vi "Parse IMU Data.vi"(6 "Packet":u8[](array[numeric]), 8 "ID":u8) -> (0 "VerticalSpeedIndicator":picture, 1 "Altitude  (/10000)":dbl, 2 "ArtificialHorizon":picture, 3 "Heading Digital":dbl format="%.1f", 4 "AltitudeIndicator":picture, 5 "CompassGauge":picture, 7 "VerticalSpeedDigital":dbl format="%.1f")   [LabVIEW 2023]
uses:
  SBG Data Cluster.ctl
panel:
  in  "ScaleUnit(F=m; T=feet)":bool
  out "output cluster":T1
  in  "Tab Control":T2(tab)
  out "Up Time":u32
  out "time stamp01":u32
  out "General Status":T3
  out "COM Status":T4
  out "Aiding Status":T5
  out "Clock Status":T6
  out "time stamp02":u32
  out "Year":u16
  out "Month":u8
  out "Day":u8
  out "Hour":u8
  out "Min":u8
  out "Sec":u8
  out "NanoSec":u32
  out "GPS TOW":u32
  out "time stamp03":u32
  out "Filtered Acc-x":sgl
  out "Filtered Acc-y":sgl
  out "Filtered Acc-z":sgl
  out "Filtered Gyro-x":sgl
  out "Filtered Gyro-y":sgl
  out "Filtered Gyro-z":sgl
  out "Temp":sgl
  out "IMU Status":T7
  out "Mag Status":T8
  out "time stamp04":u32
  out "MAG X":sgl
  out "MAG Y":sgl
  out "MAG Z":sgl
  out "ACC X":sgl
  out "ACC Y":sgl
  out "ACC Z":sgl
  out "Yaw":sgl
  out "Pitch":sgl
  out "Roll":sgl
  out "time stamp06":u32
  out "Roll Accuracy":sgl
  out "Yaw Accuracy":sgl
  out "Pitch Accuracy":sgl
  out "Internal Kalman Filter Status":T9
  out "time stamp07":u32
  out "Q0":sgl
  out "Q1":sgl
  out "Q2":sgl
  out "Q3":sgl
  out "Yaw Accuracy":sgl
  out "Pitch Accuracy":sgl
  out "Roll Accuracy":sgl
  out "EKF Latitude":dbl format="%#_16g"
  out "EKF Longitude":dbl format="%#_16g"
  out "EKF Altitude MSL":dbl format="%#_16g"
  out "time stamp08":u32
  out "EKF Velocity N":sgl
  out "EKF Velocity E":sgl
  out "EKF Velocity D":sgl
  out "EKF Velocity N Accuracy":sgl
  out "EKF Velocity E Accuracy":sgl
  out "EKF Velocity D Accuracy":sgl
  out "EKF Latitude Accuracy":sgl
  out "EKF Longitude Accuracy":sgl
  out "EKF Altitude Accuracy":sgl
  out "Undulation":sgl
  out "EKF Altitude WGS-84":dbl format="%#_16g"
  out "Ship Motion Status":T10
  out "Heave Period":sgl
  out "time stamp09":u32
  out "Heave (positive down)":sgl
  out "Surge (positive forward)":sgl
  out "Sway (positive right)":sgl
  out "Longitudinal acceleration (positive forward)":sgl
  out "Lateral acceleration (positive right)":sgl
  out "Vertical acceleration (positive down)":sgl
  out "Longitudinal velocity (positive forward)":sgl
  out "Lateral velocity (positive right)":sgl
  out "Vertical velocity (positive down)":sgl
  out "time stamp13":u32
  out "GPS1 VEL N":sgl
  out "GPS1 VEL E":sgl
  out "GPS1 VEL D":sgl
  out "GPS1 Velocity Status":string
  out "GPS1 VEL N Accuracy":sgl
  out "GPS1 VEL E Accuracy":sgl
  out "GPS1 VEL D Accuracy":sgl
  out "GPS1 TOW":u32
  out "GPS1 Course":sgl
  out "GPS1 Course Accuracy":sgl
  out "GPS1 Velocity Type":string
  out "time stamp14":u32
  out "GPS1 Base Station ID":u16
  out "GPS1 Differential Data age":u16
  out "GPS1 Altitude WGS-84 2":dbl
  out "GPS1 POS Status":string
  out "GPS1 POS Type":string
  out "GPS1 POS TOW":u32
  out "GPS1 Latitude":dbl format="%#_16g"
  out "GPS1 Longitude":dbl format="%#_16g"
  out "GPS1 Altitude MSL":dbl
  out "GPS1 Undulation":sgl
  out "GPS1 Latitude Accuracy":sgl
  out "GPS1 Longitude Accuracy":sgl
  out "GPS1 Altitude Accuracy":sgl
  out "GPS1 SV_NUM":u8
  out "GPS1 Status":T11
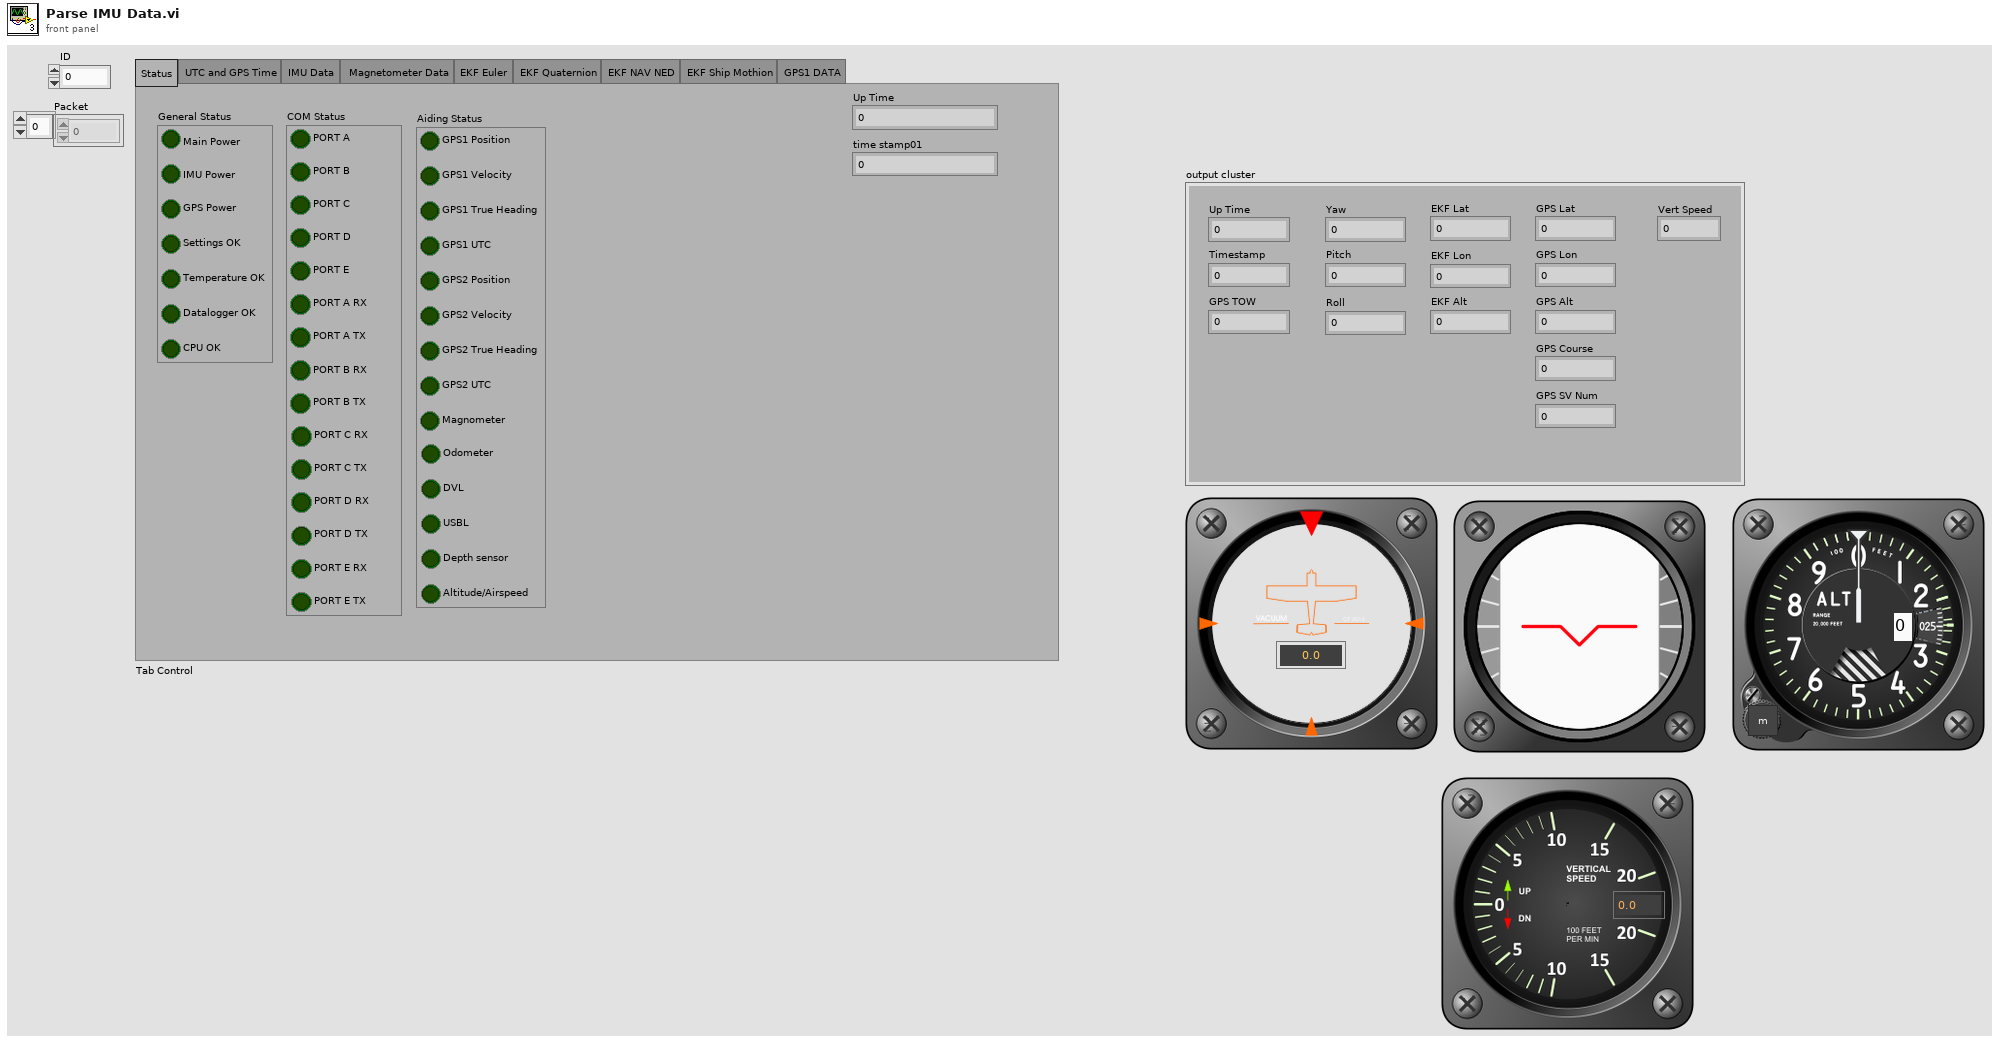
[diagram p1: front panel]
types:
  T1 = typedef "SBG Data Cluster.ctl" = cluster{"Up Time":u32, "Timestamp":u32, "Yaw":sgl, "Pitch":sgl, "Roll":sgl, "EKF Lat":dbl, "EKF Lon":dbl, "EKF Alt":dbl, "GPS Lat":dbl, "GPS Lon":dbl, "GPS Alt":dbl, "GPS Course":sgl, "GPS SV Num":u8, "GPS TOW":u32, "Vert Speed":dbl}
  T2 = enum32{"Status", "UTC and GPS Time", "IMU Data", "Magnetometer Data ", "EKF Euler", "EKF Quaternion", "EKF NAV NED", "EKF Ship Mothion", "GPS1 DATA"}
  T3 = cluster{"Main Power":bool, "IMU Power":bool, "GPS Power":bool, "Settings OK":bool, "Temperature OK":bool, "Datalogger OK":bool, "CPU OK":bool}
  T4 = cluster{"PORT A":bool, "PORT B":bool, "PORT C":bool, "PORT D":bool, "PORT E":bool, "PORT A RX":bool, "PORT A TX":bool, "PORT B RX":bool, "PORT B TX":bool, "PORT C RX":bool, "PORT C TX":bool, "PORT D RX":bool, "PORT D TX":bool, "PORT E RX":bool, "PORT E TX":bool}
  T5 = cluster{"GPS1 Position":bool, "GPS1 Velocity":bool, "GPS1 True Heading":bool, "GPS1 UTC":bool, "GPS2 Position":bool, "GPS2 Velocity":bool, "GPS2 True Heading":bool, "GPS2 UTC":bool, "Magnometer":bool, "Odometer":bool, "DVL":bool, "USBL":bool, "Depth sensor":bool, "Altitude/Airspeed":bool}
  T6 = cluster{"Clock Stable":bool, "Clock Error":bool, "Free Running":bool, "Steering":bool, "Valid and converged":bool, "UTC Sync":bool, "UTC Invalid":bool, "UTC no leap sec":bool, "UTC Valid":bool}
  T7 = cluster{"IMU COM":bool, "IMU BIT":bool, "ACC X BIT":bool, "ACC Y BIT":bool, "ACC Z BIT":bool, "GYRO X BIT":bool, "GYRO Y BIT":bool, "GYTO Z BIT":bool, "ACC  Range":bool, "GYRO Range":bool}
  T8 = cluster{"MAG X BIT":bool, "MAG Y BIT":bool, "MAG Z BIT":bool, "MAG ACC X BIT":bool, "MAG ACC Y BIT":bool, "MAG ACC Z BIT":bool, "MAG Range":bool, "MAG ACC Range":bool, "MAG Calibration":bool}
  T9 = cluster{"Mode Unintialized":bool, "Mode Vertical Gyro":bool, "Mode AHRS":bool, "Mode NAV_VEL":bool, "Attitude":bool, "Heading":bool, "Velocity":bool, "Position":bool, "Vertical Ref Used":bool, "MAG Ref Used":bool, "GPS1 VEL Used":bool, "GPS1 POS Used":bool, "Boolean array[25]":bool, "GPS1 HDT Used":bool, "GPS2 VEL Used":bool, "GPS2 POS Used":bool, "Boolean array[26]":bool, "GPS2 HDT Used":bool, "Odometer Used":bool, "DVL BT Used":bool, "DVL WT Used":bool, "Boolean array[28]":bool, "Boolean array[27]":bool, "Boolean array[28] 2":bool, "USBL Used":bool, "Air Data Used":bool, "ZUPT Used":bool, "Align Used":bool, "Depth Used":bool}
  T10 = cluster{"Heave Valid":bool, "VEL Aided":bool, "Surge Sway Included":bool, "Period Included":bool, "Period Valid":bool, "Swell Mode":bool}
  T11 = cluster{"GPS L1":bool, "GPS L2":bool, "GPS L5":bool, "GLONASS L1":bool, "GLONASS L2":bool, "GLONASS L3":bool, "Galileo E1":bool, "Galileo E5a":bool, "Galileo E5b":bool, "Galileo E5":bool, "Galileo E6":bool, "BeiDou B1":bool, "BeiDou B2":bool, "BeiDou B3":bool, "QZSS L1CA":bool, "QZSS L2C":bool, "QZSS L5":bool}
  T12 = enum16{"GPS Altitude", "Baro absolute Altitude", "Baro Vario"}
  T13 = cluster{"Boolean array[0]":bool, "Boolean array[1]":bool, "Boolean array[2]":bool, "Boolean array[3]":bool, "Boolean array[4]":bool, "Boolean array[5]":bool, "Boolean array[6]":bool, "Boolean array[7]":bool, "Boolean array[8]":bool, "Boolean array[9]":bool, "Boolean array[10]":bool, "Boolean array[11]":bool, "Boolean array[12]":bool, "Boolean array[13]":bool, "Boolean array[14]":bool}
  T14 = cluster{"Boolean array[0]":bool, "Boolean array[1]":bool, "Boolean array[2]":bool, "Boolean array[3]":bool, "Boolean array[4]":bool, "Boolean array[5]":bool, "Boolean array[6]":bool, "Boolean array[7]":bool, "Boolean array[8]":bool, "Boolean array[9]":bool, "Boolean array[10]":bool, "Boolean array[11]":bool, "Boolean array[12]":bool, "Boolean array[13]":bool}
  T15 = cluster{"Boolean array[0]":bool, "Boolean array[1]":bool, "Boolean array[2]":bool, "Boolean array[3]":bool, "Boolean array[4]":bool, "Boolean array[5]":bool, "Boolean array[6]":bool}
  T16 = cluster{"Boolean array[0]":bool, "Boolean array[1]":bool, "Boolean array[2]":bool, "Boolean array[3]":bool, "Boolean array[4]":bool, "Boolean array[5]":bool, "Boolean array[6]":bool, "Boolean array[7]":bool, "Boolean array[8]":bool}
  T17 = cluster{"Boolean array[0]":bool, "Boolean array[1]":bool, "Boolean array[2]":bool, "Boolean array[3]":bool, "Boolean array[4]":bool, "Boolean array[5]":bool, "Boolean array[6]":bool, "Boolean array[7]":bool, "Boolean array[8]":bool, "Boolean array[9]":bool}
  T18 = cluster{"Boolean array[0]":bool, "Boolean array[1]":bool, "Boolean array[2]":bool, "Boolean array[3]":bool, "Boolean array[4]":bool, "Boolean array[5]":bool, "Boolean array[6]":bool, "Boolean array[7]":bool, "Boolean array[8]":bool, "Boolean array[9]":bool, "Boolean array[10]":bool, "Boolean array[11]":bool, "Boolean array[12]":bool, "Boolean array[13]":bool, "Boolean array[14]":bool, "Boolean array[15]":bool, "Boolean array[16]":bool, "Boolean array[17]":bool, "Boolean array[18]":bool, "Boolean array[19]":bool, "Boolean array[20]":bool, "Boolean array[21]":bool, "Boolean array[22]":bool, "Boolean array[23]":bool, "Boolean array[24]":bool, "Boolean array[25]":bool, "Boolean array[26]":bool, "Boolean array[27]":bool, "Boolean array[28]":bool}
  T19 = cluster{"Boolean array[0]":bool, "Boolean array[1]":bool, "Boolean array[2]":bool, "Boolean array[3]":bool, "Boolean array[4]":bool, "Boolean array[5]":bool}
  T20 = cluster{"Boolean array[0]":bool, "Boolean array[1]":bool, "Boolean array[2]":bool, "Boolean array[3]":bool, "Boolean array[4]":bool, "Boolean array[5]":bool, "Boolean array[6]":bool, "Boolean array[7]":bool, "Boolean array[8]":bool, "Boolean array[9]":bool, "Boolean array[10]":bool, "Boolean array[11]":bool, "Boolean array[12]":bool, "Boolean array[13]":bool, "Boolean array[14]":bool, "Boolean array[15]":bool, "Boolean array[16]":bool}
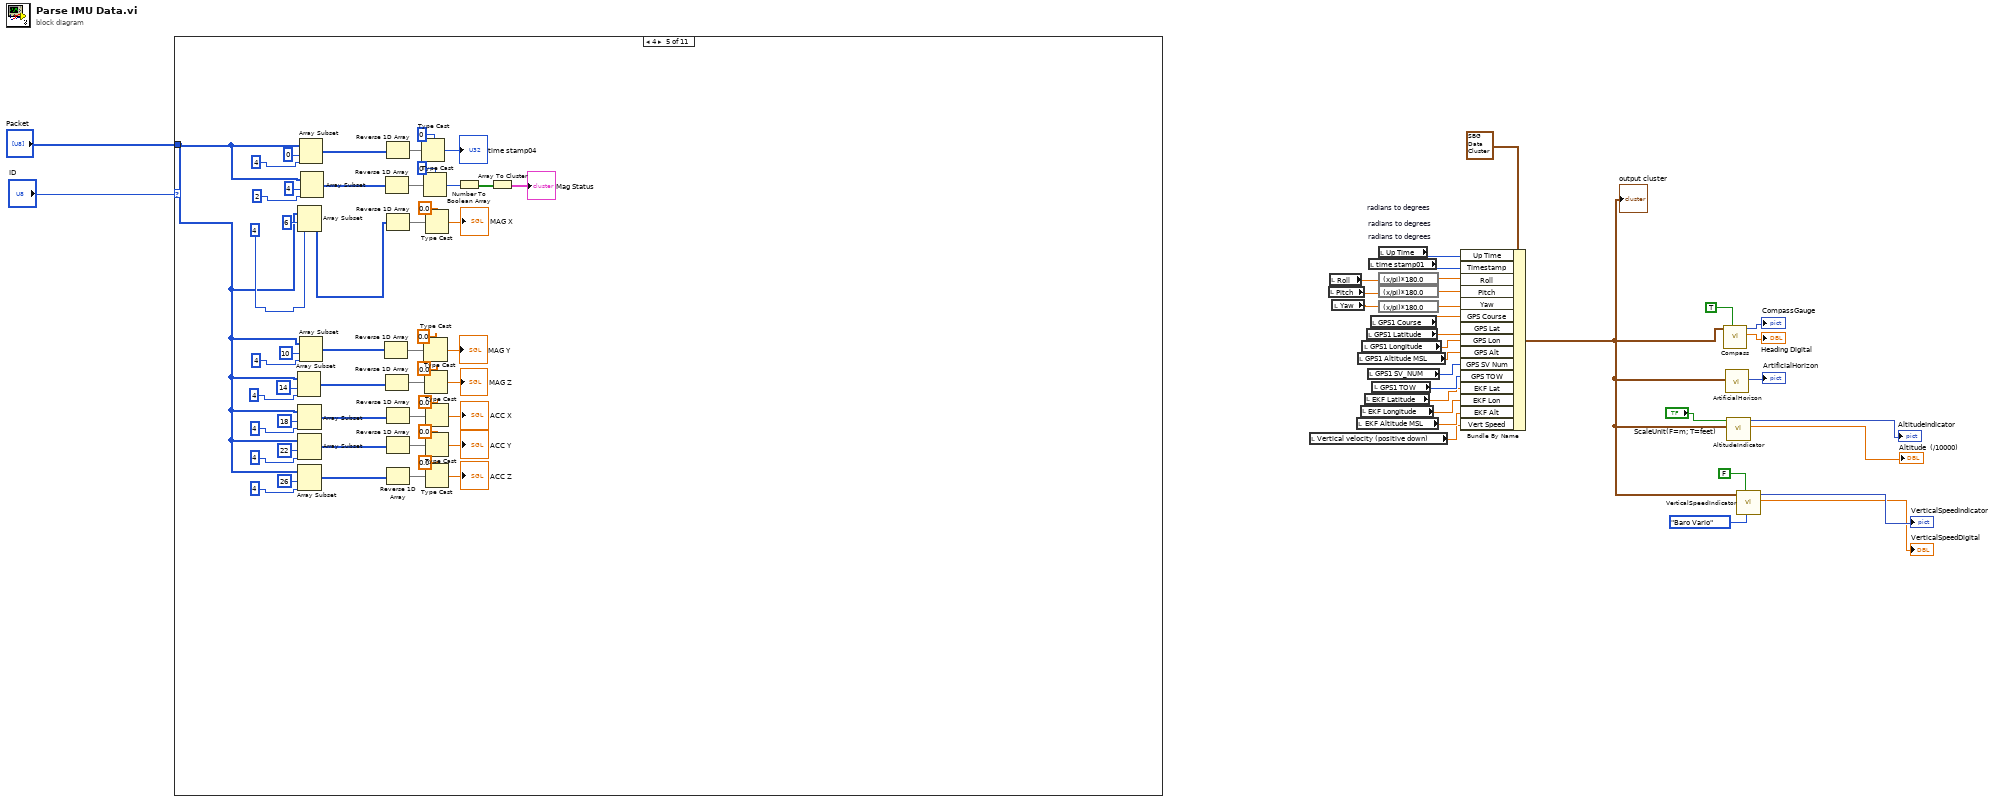
[diagram p0: block diagram]
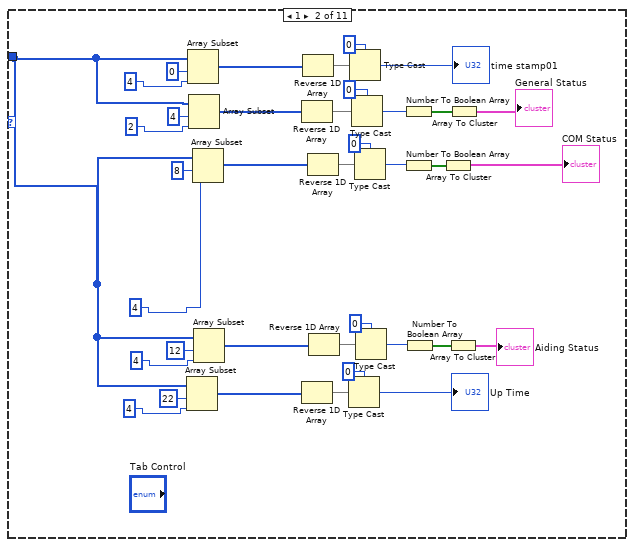
[diagram p3: hidden frame]
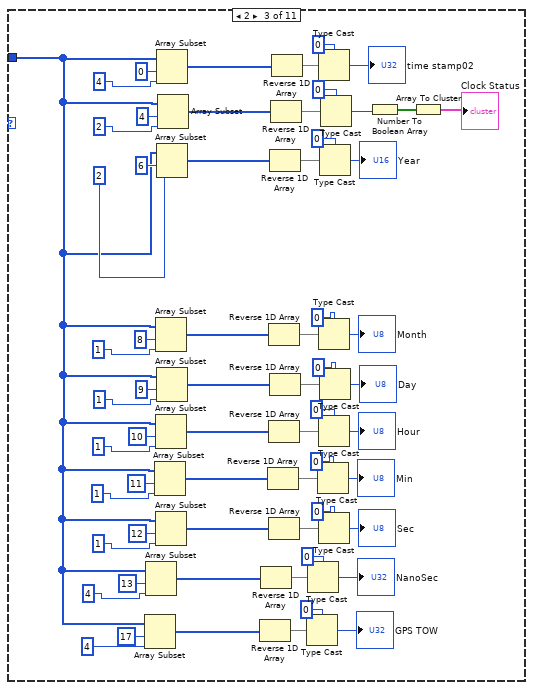
[diagram p4: hidden frame]
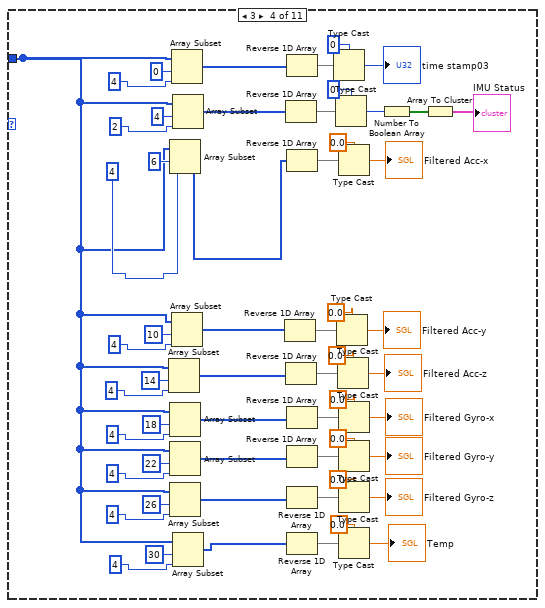
[diagram p5: hidden frame]
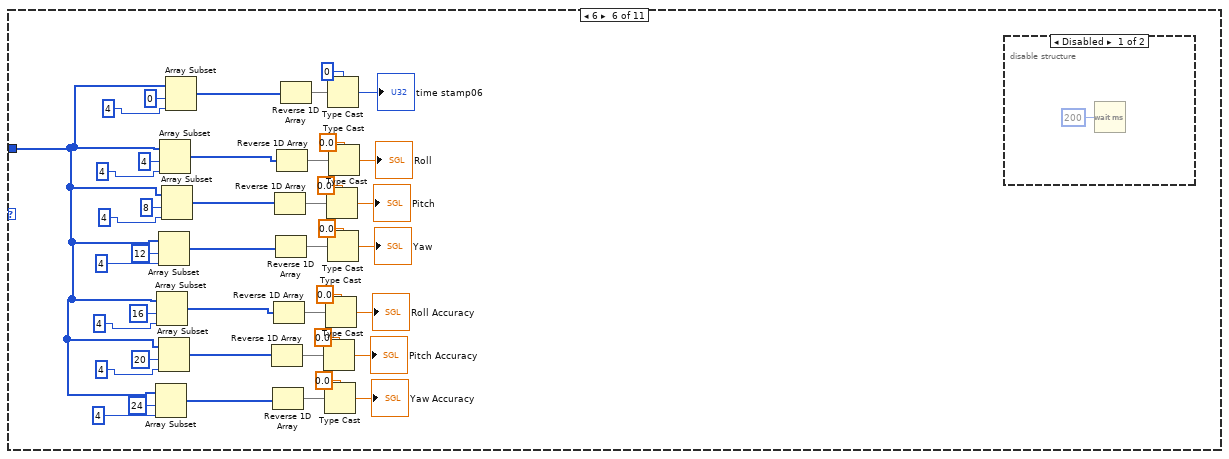
[diagram p6: hidden frame]
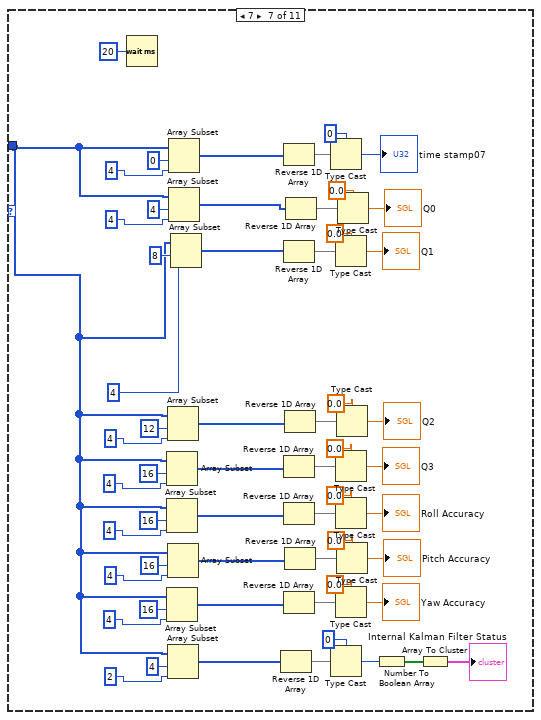
[diagram p8: hidden frame]
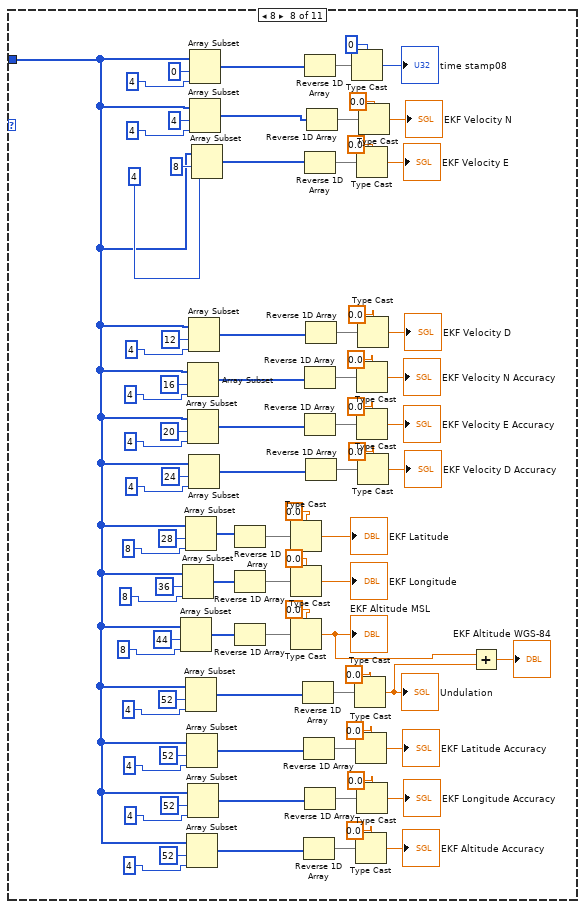
[diagram p9: hidden frame]
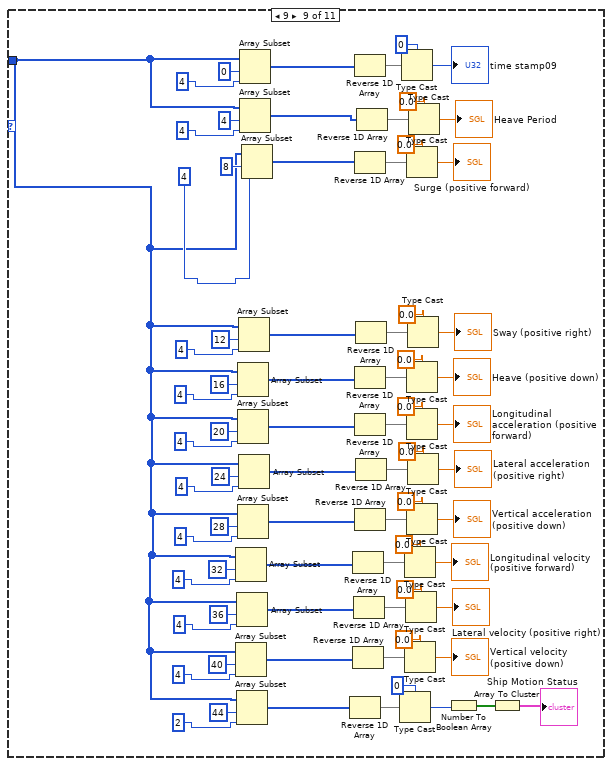
[diagram p10: hidden frame]
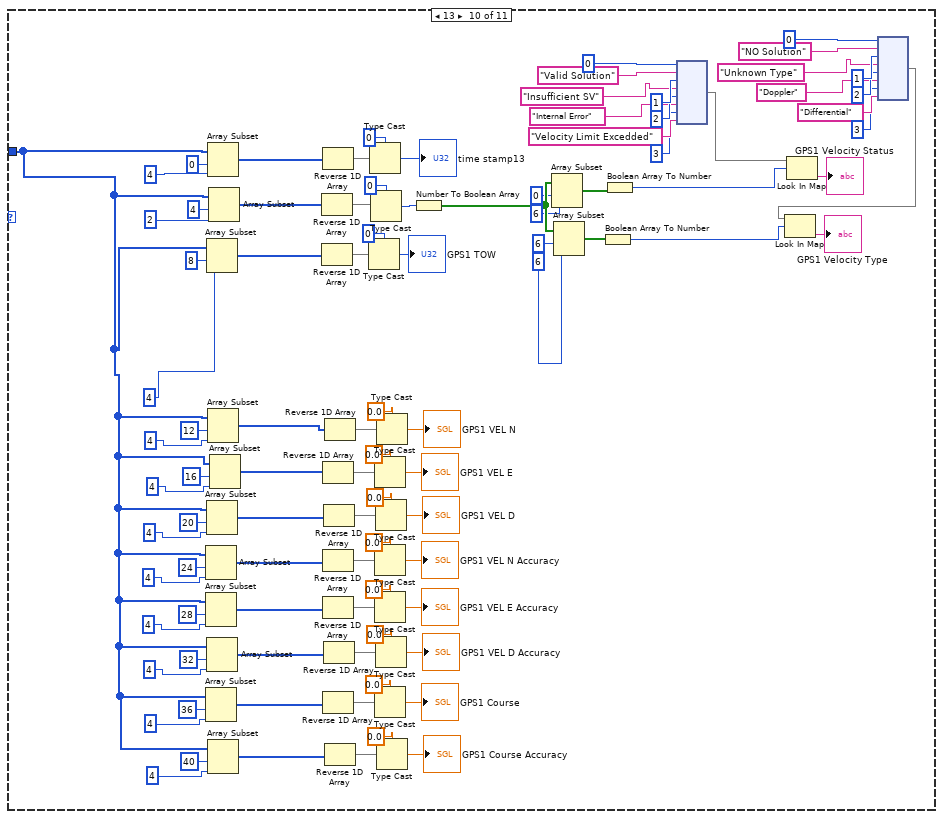
[diagram p11: hidden frame]
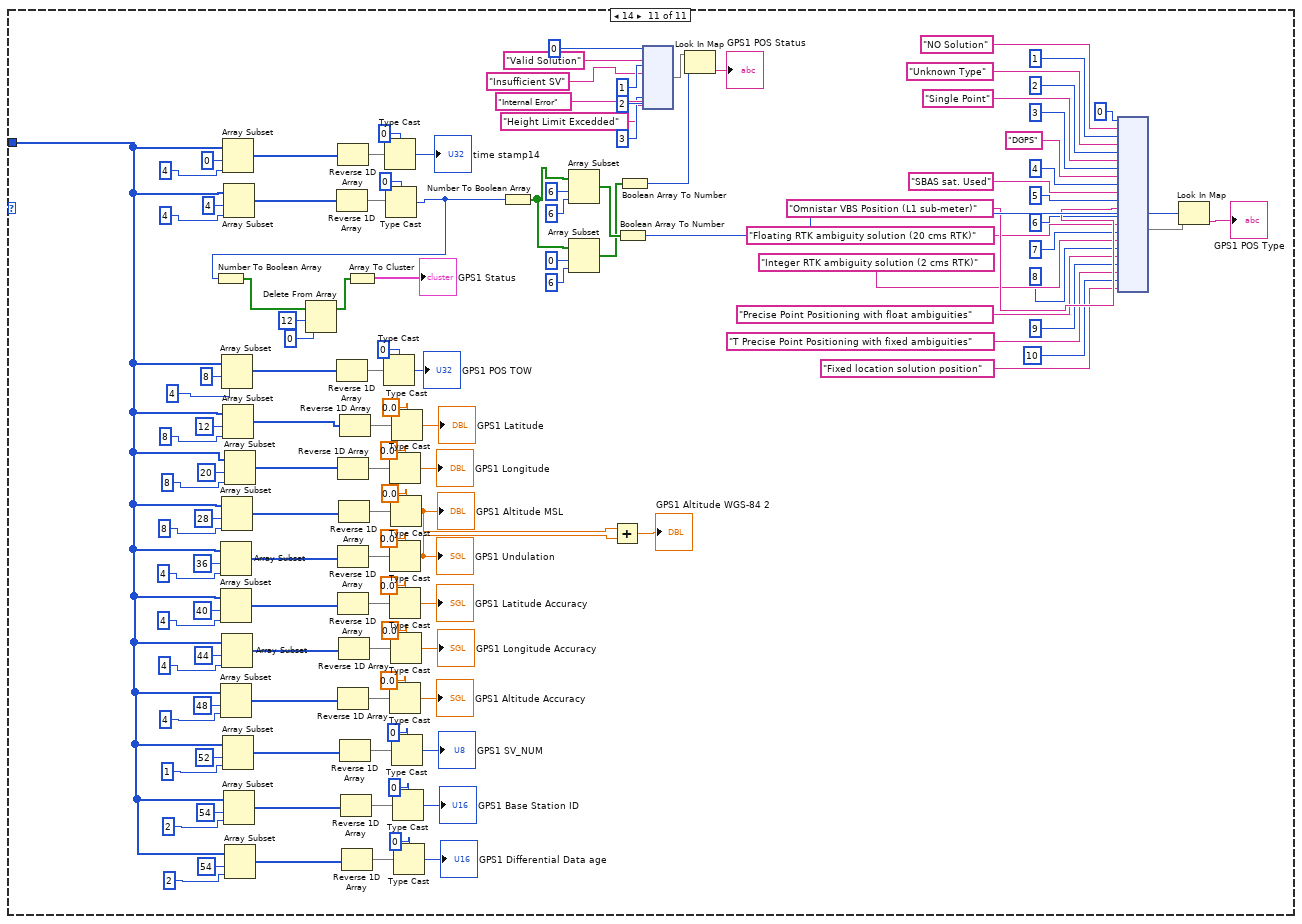
[diagram p12: hidden frame]
diagram:
  n1 = case shown="4" "ID" {
    tunnel: "Packet" -> [_ w37 w71 w137 w191 w246 w287 w344 w430 w539 w610]
    frame 0, Default {
    }
    frame 1 {
      n2 = Array Subset(array=w37, index=22, length=4) -> (w39:u8[])
      n3 = Array Subset(array=w37, index=0, length=4) -> (w68:u8[])
      n4 = Array Subset(array=w37, index=4, length=2) -> (w66:u8[])
      n5 = Array Subset(array=w37, index=8, length=4) -> (w54:u8[])
      n6 = Array Subset(array=w37, index=12, length=4) -> (w47:u8[])
      n7 = Reverse 1D Array(array=w66) -> (reversed array=w70:u8[])
      n8 = Reverse 1D Array(array=w39) -> (reversed array=w38:u8[])
      n9 = Reverse 1D Array(array=w68) -> (reversed array=w69:u8[])
      n10 = Reverse 1D Array(array=w54) -> (reversed array=w53:u8[])
      n11 = Reverse 1D Array(array=w47) -> (reversed array=w48:u8[])
      n12 = Type Cast(type=u32 0, x=w38) -> (*(type *) &x=→"Up Time":u32)
      n13 = Type Cast(type=u32 0, x=w69) -> (*(type *) &x=→"time stamp01":u32)
      n14 = Type Cast(type=u16 0, x=w70) -> (*(type *) &x=w59:u16)
      n15 = Type Cast(type=u32 0, x=w53) -> (*(type *) &x=w52:u32)
      n16 = Type Cast(type=u32 0, x=w48) -> (*(type *) &x=w49:u32)
      n17 = Number To Boolean Array(number=w59) -> (Boolean array=w58:bool[])
      n18 = Number To Boolean Array(number=w52) -> (Boolean array=w51:bool[])
      n19 = Number To Boolean Array(number=w49) -> (Boolean array=w50:bool[])
      n20 = Array To Cluster(array=w51) -> (cluster=→"COM Status":T13)
      n21 = Array To Cluster(array=w50) -> (cluster=→"Aiding Status":T14)
      n22 = Array To Cluster(array=w58) -> (cluster=→"General Status":T15)
    }
    frame 2 {
      n23 = Array Subset(array=w71, index=17, length=4) -> (w73:u8[])
      n24 = Array Subset(array=w71, index=13, length=4) -> (w82:u8[])
      n25 = Array Subset(array=w71, index=11, length=1) -> (w94:u8[])
      n26 = Array Subset(array=w71, index=8, length=1) -> (w109:u8[])
      n27 = Array Subset(array=w71, index=10, length=1) -> (w85:u8[])
      n28 = Array Subset(array=w71, index=12, length=1) -> (w97:u8[])
      n29 = Array Subset(array=w71, index=0, length=4) -> (w125:u8[])
      n30 = Array Subset(array=w71, index=6, length=2) -> (w118:u8[])
      n31 = Array Subset(array=w71, index=9, length=1) -> (w106:u8[])
      n32 = Array Subset(array=w71, index=4, length=2) -> (w128:u8[])
      n33 = Reverse 1D Array(array=w73) -> (reversed array=w72:u8[])
      n34 = Reverse 1D Array(array=w82) -> (reversed array=w83:u8[])
      n35 = Reverse 1D Array(array=w94) -> (reversed array=w95:u8[])
      n36 = Reverse 1D Array(array=w109) -> (reversed array=w108:u8[])
      n37 = Reverse 1D Array(array=w85) -> (reversed array=w84:u8[])
      n38 = Reverse 1D Array(array=w97) -> (reversed array=w96:u8[])
      n39 = Reverse 1D Array(array=w118) -> (reversed array=w119:u8[])
      n40 = Reverse 1D Array(array=w106) -> (reversed array=w107:u8[])
      n41 = Reverse 1D Array(array=w128) -> (reversed array=w123:u8[])
      n42 = Reverse 1D Array(array=w125) -> (reversed array=w124:u8[])
      n43 = Type Cast(type=u32 0, x=w72) -> (*(type *) &x=→"GPS TOW":u32)
      n44 = Type Cast(type=u32 0, x=w83) -> (*(type *) &x=→"NanoSec":u32)
      n45 = Type Cast(type=u8 0, x=w95) -> (*(type *) &x=→"Min":u8)
      n46 = Type Cast(type=u32 0, x=w124) -> (*(type *) &x=→"time stamp02":u32)
      n47 = Type Cast(type=u8 0, x=w108) -> (*(type *) &x=→"Month":u8)
      n48 = Type Cast(type=u8 0, x=w84) -> (*(type *) &x=→"Hour":u8)
      n49 = Type Cast(type=u8 0, x=w96) -> (*(type *) &x=→"Sec":u8)
      n50 = Type Cast(type=u16 0, x=w119) -> (*(type *) &x=→"Year":u16)
      n51 = Type Cast(type=u8 0, x=w107) -> (*(type *) &x=→"Day":u8)
      n52 = Type Cast(type=u16 0, x=w123) -> (*(type *) &x=w120:u16)
      n53 = Number To Boolean Array(number=w120) -> (Boolean array=w122:bool[])
      n54 = Array To Cluster(array=w122) -> (cluster=→"Clock Status":T16)
    }
    frame 3 {
      n55 = Array Subset(array=w137, index=14, length=4) -> (w156:u8[])
      n56 = Array Subset(array=w137, index=6, length=4) -> (w164:u8[])
      n57 = Array Subset(array=w137, index=18, length=4) -> (w155:u8[])
      n58 = Array Subset(array=w137, index=22, length=4) -> (w144:u8[])
      n59 = Array Subset(array=w137, index=26, length=4) -> (w143:u8[])
      n60 = Array Subset(array=w137, index=0, length=4) -> (w171:u8[])
      n61 = Array Subset(array=w137, index=10, length=4) -> (w160:u8[])
      n62 = Array Subset(array=w137, index=4, length=2) -> (w174:u8[])
      n63 = Array Subset(array=w137, index=30, length=4) -> (w176:u8[])
      n64 = Reverse 1D Array(array=w160) -> (reversed array=w163:u8[])
      n65 = Reverse 1D Array(array=w174) -> (reversed array=w168:u8[])
      n66 = Reverse 1D Array(array=w156) -> (reversed array=w157:u8[])
      n67 = Reverse 1D Array(array=w171) -> (reversed array=w169:u8[])
      n68 = Reverse 1D Array(array=w164) -> (reversed array=w165:u8[])
      n69 = Reverse 1D Array(array=w155) -> (reversed array=w154:u8[])
      n70 = Reverse 1D Array(array=w144) -> (reversed array=w145:u8[])
      n71 = Reverse 1D Array(array=w143) -> (reversed array=w142:u8[])
      n72 = Reverse 1D Array(array=w176) -> (reversed array=w170:u8[])
      n73 = Type Cast(type=u32 0, x=w169) -> (*(type *) &x=→"time stamp03":u32)
      n74 = Type Cast(type=u16 0, x=w168) -> (*(type *) &x=w134:u16)
      n75 = Type Cast(type=sgl 0.0, x=w163) -> (*(type *) &x=→"Filtered Acc-y":sgl)
      n76 = Type Cast(type=sgl 0.0, x=w157) -> (*(type *) &x=→"Filtered Acc-z":sgl)
      n77 = Type Cast(type=sgl 0.0, x=w165) -> (*(type *) &x=→"Filtered Acc-x":sgl)
      n78 = Type Cast(type=sgl 0.0, x=w154) -> (*(type *) &x=→"Filtered Gyro-x":sgl)
      n79 = Type Cast(type=sgl 0.0, x=w145) -> (*(type *) &x=→"Filtered Gyro-y":sgl)
      n80 = Type Cast(type=sgl 0.0, x=w142) -> (*(type *) &x=→"Filtered Gyro-z":sgl)
      n81 = Type Cast(type=sgl 0.0, x=w170) -> (*(type *) &x=→"Temp":sgl)
      n82 = Number To Boolean Array(number=w134) -> (Boolean array=w136:bool[])
      n83 = Array To Cluster(array=w136) -> (cluster=→"IMU Status":T17)
    }
    frame 4 {
      n84 = Array Subset(array=w191, index=14, length=4) -> (w213:u8[])
      n85 = Array Subset(array=w191, index=6, length=4) -> (w221:u8[])
      n86 = Array Subset(array=w191, index=18, length=4) -> (w212:u8[])
      n87 = Array Subset(array=w191, index=22, length=4) -> (w201:u8[])
      n88 = Array Subset(array=w191, index=26, length=4) -> (w200:u8[])
      n89 = Array Subset(array=w191, index=0, length=4) -> (w227:u8[])
      n90 = Array Subset(array=w191, index=10, length=4) -> (w217:u8[])
      n91 = Array Subset(array=w191, index=4, length=2) -> (w230:u8[])
      n92 = Reverse 1D Array(array=w217) -> (reversed array=w220:u8[])
      n93 = Reverse 1D Array(array=w230) -> (reversed array=w225:u8[])
      n94 = Reverse 1D Array(array=w213) -> (reversed array=w214:u8[])
      n95 = Reverse 1D Array(array=w227) -> (reversed array=w226:u8[])
      n96 = Reverse 1D Array(array=w221) -> (reversed array=w222:u8[])
      n97 = Reverse 1D Array(array=w212) -> (reversed array=w211:u8[])
      n98 = Reverse 1D Array(array=w201) -> (reversed array=w202:u8[])
      n99 = Reverse 1D Array(array=w200) -> (reversed array=w199:u8[])
      n100 = Type Cast(type=u32 0, x=w226) -> (*(type *) &x=→"time stamp04":u32)
      n101 = Type Cast(type=u16 0, x=w225) -> (*(type *) &x=w192:u16)
      n102 = Type Cast(type=sgl 0.0, x=w220) -> (*(type *) &x=→"MAG Y":sgl)
      n103 = Type Cast(type=sgl 0.0, x=w214) -> (*(type *) &x=→"MAG Z":sgl)
      n104 = Type Cast(type=sgl 0.0, x=w222) -> (*(type *) &x=→"MAG X":sgl)
      n105 = Type Cast(type=sgl 0.0, x=w211) -> (*(type *) &x=→"ACC X":sgl)
      n106 = Type Cast(type=sgl 0.0, x=w202) -> (*(type *) &x=→"ACC Y":sgl)
      n107 = Type Cast(type=sgl 0.0, x=w199) -> (*(type *) &x=→"ACC Z":sgl)
      n108 = Number To Boolean Array(number=w192) -> (Boolean array=w194:bool[])
      n109 = Array To Cluster(array=w194) -> (cluster=→"Mag Status":T16)
    }
    frame 6 {
      n110 = Array Subset(array=w246, index=24, length=4) -> (w252:u8[])
      n111 = Array Subset(array=w246, index=16, length=4) -> (w260:u8[])
      n112 = Array Subset(array=w246, index=12, length=4) -> (w270:u8[])
      n113 = Array Subset(array=w246, index=20, length=4) -> (w256:u8[])
      n114 = Array Subset(array=w246, index=4, length=4) -> (w276:u8[])
      n115 = Array Subset(array=w246, index=8, length=4) -> (w273:u8[])
      n116 = Array Subset(array=w246, index=0, length=4) -> (w248:u8[])
      n117 = Reverse 1D Array(array=w256) -> (reversed array=w259:u8[])
      n118 = Reverse 1D Array(array=w252) -> (reversed array=w253:u8[])
      n119 = Reverse 1D Array(array=w260) -> (reversed array=w261:u8[])
      n120 = Reverse 1D Array(array=w273) -> (reversed array=w275:u8[])
      n121 = Reverse 1D Array(array=w270) -> (reversed array=w271:u8[])
      n122 = Reverse 1D Array(array=w276) -> (reversed array=w277:u8[])
      n123 = Reverse 1D Array(array=w248) -> (reversed array=w247:u8[])
      n124 = Type Cast(type=sgl 0.0, x=w259) -> (*(type *) &x=→"Pitch Accuracy":sgl)
      n125 = Type Cast(type=sgl 0.0, x=w253) -> (*(type *) &x=→"Yaw Accuracy":sgl)
      n126 = Type Cast(type=sgl 0.0, x=w261) -> (*(type *) &x=→"Roll Accuracy":sgl)
      n127 = Type Cast(type=sgl 0.0, x=w275) -> (*(type *) &x=→"Pitch":sgl)
      n128 = Type Cast(type=u32 0, x=w247) -> (*(type *) &x=→"time stamp06":u32)
      n129 = Type Cast(type=sgl 0.0, x=w271) -> (*(type *) &x=→"Yaw":sgl)
      n130 = Type Cast(type=sgl 0.0, x=w277) -> (*(type *) &x=→"Roll":sgl)
      n131 = disable-structure shown="Disabled" {
        frame Disabled {
          n132 = Wait (ms)(milliseconds to wait=u32 200) -> ()  [unwired: 1 out]
        }
        frame Enabled {
        }
      }
    }
    frame 7 {
      n133 = Wait (ms)(milliseconds to wait=u32 20) -> ()  [unwired: 1 out]
      n134 = Array Subset(array=w287, index=16, length=4) -> (w319:u8[])
      n135 = Array Subset(array=w287, index=16, length=4) -> (w308:u8[])
      n136 = Array Subset(array=w287, index=16, length=4) -> (w296:u8[])
      n137 = Array Subset(array=w287, index=12, length=4) -> (w326:u8[])
      n138 = Array Subset(array=w287, index=16, length=4) -> (w307:u8[])
      n139 = Array Subset(array=w287, index=4, length=2) -> (w292:u8[])
      n140 = Array Subset(array=w287, index=0, length=4) -> (w324:u8[])
      n141 = Array Subset(array=w287, index=4, length=4) -> (w334:u8[])
      n142 = Array Subset(array=w287, index=8, length=4) -> (w330:u8[])
      n143 = Reverse 1D Array(array=w292) -> (reversed array=w291:u8[])
      n144 = Reverse 1D Array(array=w324) -> (reversed array=w325:u8[])
      n145 = Reverse 1D Array(array=w330) -> (reversed array=w333:u8[])
      n146 = Reverse 1D Array(array=w319) -> (reversed array=w318:u8[])
      n147 = Reverse 1D Array(array=w308) -> (reversed array=w309:u8[])
      n148 = Reverse 1D Array(array=w296) -> (reversed array=w297:u8[])
      n149 = Reverse 1D Array(array=w326) -> (reversed array=w327:u8[])
      n150 = Reverse 1D Array(array=w307) -> (reversed array=w306:u8[])
      n151 = Reverse 1D Array(array=w334) -> (reversed array=w335:u8[])
      n152 = Type Cast(type=u32 0, x=w325) -> (*(type *) &x=→"time stamp07":u32)
      n153 = Type Cast(type=u16 0, x=w291) -> (*(type *) &x=w288:u16)
      n154 = Type Cast(type=sgl 0.0, x=w333) -> (*(type *) &x=→"Q1":sgl)
      n155 = Type Cast(type=sgl 0.0, x=w318) -> (*(type *) &x=→"Q3":sgl)
      n156 = Type Cast(type=sgl 0.0, x=w309) -> (*(type *) &x=→"Roll Accuracy":sgl)
      n157 = Type Cast(type=sgl 0.0, x=w297) -> (*(type *) &x=→"Yaw Accuracy":sgl)
      n158 = Type Cast(type=sgl 0.0, x=w327) -> (*(type *) &x=→"Q2":sgl)
      n159 = Type Cast(type=sgl 0.0, x=w306) -> (*(type *) &x=→"Pitch Accuracy":sgl)
      n160 = Type Cast(type=sgl 0.0, x=w335) -> (*(type *) &x=→"Q0":sgl)
      n161 = Number To Boolean Array(number=w288) -> (Boolean array=w290:bool[])
      n162 = Array To Cluster(array=w290) -> (cluster=→"Internal Kalman Filter Status":T18)
    }
    frame 8 {
      n163 = Array Subset(array=w344, index=44, length=8) -> (w415:u8[])
      n164 = Array Subset(array=w344, index=36, length=8) -> (w416:u8[])
      n165 = Array Subset(array=w344, index=28, length=8) -> (w423:u8[])
      n166 = Array Subset(array=w344, index=52, length=4) -> (w366:u8[])
      n167 = Array Subset(array=w344, index=52, length=4) -> (w361:u8[])
      n168 = Array Subset(array=w344, index=52, length=4) -> (w349:u8[])
      n169 = Array Subset(array=w344, index=16, length=4) -> (w388:u8[])
      n170 = Array Subset(array=w344, index=20, length=4) -> (w377:u8[])
      n171 = Array Subset(array=w344, index=52, length=4) -> (w352:u8[])
      n172 = Array Subset(array=w344, index=12, length=4) -> (w395:u8[])
      n173 = Array Subset(array=w344, index=24, length=4) -> (w376:u8[])
      n174 = Array Subset(array=w344, index=0, length=4) -> (w393:u8[])
      n175 = Array Subset(array=w344, index=4, length=4) -> (w403:u8[])
      n176 = Array Subset(array=w344, index=8, length=4) -> (w399:u8[])
      n177 = Reverse 1D Array(array=w423) -> (reversed array=w421:u8[])
      n178 = Reverse 1D Array(array=w416) -> (reversed array=w414:u8[])
      n179 = Reverse 1D Array(array=w415) -> (reversed array=w413:u8[])
      n180 = Type Cast(type=0.0, x=w421) -> (*(type *) &x=→"EKF Latitude":dbl)
      n181 = Type Cast(type=0.0, x=w414) -> (*(type *) &x=→"EKF Longitude":dbl)
      n182 = Type Cast(type=0.0, x=w413) -> (*(type *) &x=w365:dbl)
      "EKF Altitude MSL" <- w365
      n183 = Reverse 1D Array(array=w366) -> (reversed array=w367:u8[])
      n184 = Reverse 1D Array(array=w361) -> (reversed array=w360:u8[])
      n185 = Reverse 1D Array(array=w349) -> (reversed array=w348:u8[])
      n186 = Reverse 1D Array(array=w393) -> (reversed array=w394:u8[])
      n187 = Reverse 1D Array(array=w399) -> (reversed array=w402:u8[])
      n188 = Reverse 1D Array(array=w388) -> (reversed array=w387:u8[])
      n189 = Reverse 1D Array(array=w377) -> (reversed array=w378:u8[])
      n190 = Reverse 1D Array(array=w352) -> (reversed array=w353:u8[])
      n191 = Reverse 1D Array(array=w395) -> (reversed array=w396:u8[])
      n192 = Reverse 1D Array(array=w376) -> (reversed array=w375:u8[])
      n193 = Reverse 1D Array(array=w403) -> (reversed array=w404:u8[])
      n194 = Type Cast(type=u32 0, x=w394) -> (*(type *) &x=→"time stamp08":u32)
      n195 = Type Cast(type=sgl 0.0, x=w367) -> (*(type *) &x=w364:sgl)
      "Undulation" <- w364
      n196 = Type Cast(type=sgl 0.0, x=w360) -> (*(type *) &x=→"EKF Latitude Accuracy":sgl)
      n197 = Type Cast(type=sgl 0.0, x=w348) -> (*(type *) &x=→"EKF Altitude Accuracy":sgl)
      n198 = Type Cast(type=sgl 0.0, x=w402) -> (*(type *) &x=→"EKF Velocity E":sgl)
      n199 = Type Cast(type=sgl 0.0, x=w387) -> (*(type *) &x=→"EKF Velocity N Accuracy":sgl)
      n200 = Type Cast(type=sgl 0.0, x=w378) -> (*(type *) &x=→"EKF Velocity E Accuracy":sgl)
      n201 = Type Cast(type=sgl 0.0, x=w353) -> (*(type *) &x=→"EKF Longitude Accuracy":sgl)
      n202 = Type Cast(type=sgl 0.0, x=w396) -> (*(type *) &x=→"EKF Velocity D":sgl)
      n203 = Type Cast(type=sgl 0.0, x=w375) -> (*(type *) &x=→"EKF Velocity D Accuracy":sgl)
      n204 = Type Cast(type=sgl 0.0, x=w404) -> (*(type *) &x=→"EKF Velocity N":sgl)
      n205 = Add(x=w365, y=w364) -> (x+y=→"EKF Altitude WGS-84":dbl)
    }
    frame 9 {
      n206 = Array Subset(array=w430, index=32, length=4) -> (w446:u8[])
      n207 = Array Subset(array=w430, index=40, length=4) -> (w455:u8[])
      n208 = Array Subset(array=w430, index=36, length=4) -> (w445:u8[])
      n209 = Array Subset(array=w430, index=44, length=2) -> (w435:u8[])
      n210 = Array Subset(array=w430, index=16, length=4) -> (w496:u8[])
      n211 = Array Subset(array=w430, index=20, length=4) -> (w501:u8[])
      n212 = Array Subset(array=w430, index=28, length=4) -> (w462:u8[])
      n213 = Array Subset(array=w430, index=12, length=4) -> (w492:u8[])
      n214 = Array Subset(array=w430, index=24, length=4) -> (w502:u8[])
      n215 = Array Subset(array=w430, index=0, length=4) -> (w494:u8[])
      n216 = Array Subset(array=w430, index=4, length=4) -> (w486:u8[])
      n217 = Array Subset(array=w430, index=8, length=4) -> (w489:u8[])
      n218 = Reverse 1D Array(array=w435) -> (reversed array=w434:u8[])
      n219 = Reverse 1D Array(array=w446) -> (reversed array=w447:u8[])
      n220 = Reverse 1D Array(array=w455) -> (reversed array=w456:u8[])
      n221 = Reverse 1D Array(array=w445) -> (reversed array=w444:u8[])
      n222 = Reverse 1D Array(array=w494) -> (reversed array=w493:u8[])
      n223 = Reverse 1D Array(array=w489) -> (reversed array=w487:u8[])
      n224 = Reverse 1D Array(array=w496) -> (reversed array=w497:u8[])
      n225 = Reverse 1D Array(array=w501) -> (reversed array=w500:u8[])
      n226 = Reverse 1D Array(array=w462) -> (reversed array=w461:u8[])
      n227 = Reverse 1D Array(array=w492) -> (reversed array=w491:u8[])
      n228 = Reverse 1D Array(array=w502) -> (reversed array=w503:u8[])
      n229 = Reverse 1D Array(array=w486) -> (reversed array=w485:u8[])
      n230 = Type Cast(type=u16 0, x=w434) -> (*(type *) &x=w431:u16)
      n231 = Type Cast(type=u32 0, x=w493) -> (*(type *) &x=→"time stamp09":u32)
      n232 = Type Cast(type=sgl 0.0, x=w447) -> (*(type *) &x=→"Longitudinal velocity (positive forward)":sgl)
      n233 = Type Cast(type=sgl 0.0, x=w456) -> (*(type *) &x=→"Vertical velocity (positive down)":sgl)
      n234 = Type Cast(type=sgl 0.0, x=w444) -> (*(type *) &x=→"Lateral velocity (positive right)":sgl)
      n235 = Type Cast(type=sgl 0.0, x=w487) -> (*(type *) &x=→"Surge (positive forward)":sgl)
      n236 = Type Cast(type=sgl 0.0, x=w497) -> (*(type *) &x=→"Heave (positive down)":sgl)
      n237 = Type Cast(type=sgl 0.0, x=w500) -> (*(type *) &x=→"Longitudinal acceleration (positive forward)":sgl)
      n238 = Type Cast(type=sgl 0.0, x=w461) -> (*(type *) &x=→"Vertical acceleration (positive down)":sgl)
      n239 = Type Cast(type=sgl 0.0, x=w491) -> (*(type *) &x=→"Sway (positive right)":sgl)
      n240 = Type Cast(type=sgl 0.0, x=w503) -> (*(type *) &x=→"Lateral acceleration (positive right)":sgl)
      n241 = Type Cast(type=sgl 0.0, x=w485) -> (*(type *) &x=→"Heave Period":sgl)
      n242 = Number To Boolean Array(number=w431) -> (Boolean array=w433:bool[])
      n243 = Array To Cluster(array=w433) -> (cluster=→"Ship Motion Status":T19)
    }
    frame 13 {
      n244 = Array Subset(array=w539, index=24, length=4) -> (w578:u8[])
      n245 = Array Subset(array=w539, index=28, length=4) -> (w583:u8[])
      n246 = Array Subset(array=w539, index=36, length=4) -> (w550:u8[])
      n247 = Array Subset(array=w539, index=8, length=4) -> (w599:u8[])
      n248 = Array Subset(array=w539, index=20, length=4) -> (w577:u8[])
      n249 = Array Subset(array=w539, index=32, length=4) -> (w584:u8[])
      n250 = Array Subset(array=w539, index=0, length=4) -> (w597:u8[])
      n251 = Array Subset(array=w539, index=12, length=4) -> (w571:u8[])
      n252 = Array Subset(array=w539, index=40, length=4) -> (w541:u8[])
      n253 = Array Subset(array=w539, index=4, length=2) -> (w596:u8[])
      n254 = Array Subset(array=w539, index=16, length=4) -> (w574:u8[])
      n255 = Reverse 1D Array(array=w596) -> (reversed array=w533:u8[])
      n256 = Reverse 1D Array(array=w599) -> (reversed array=w600:u8[])
      n257 = Reverse 1D Array(array=w597) -> (reversed array=w598:u8[])
      n258 = Reverse 1D Array(array=w574) -> (reversed array=w572:u8[])
      n259 = Reverse 1D Array(array=w578) -> (reversed array=w579:u8[])
      n260 = Reverse 1D Array(array=w583) -> (reversed array=w582:u8[])
      n261 = Reverse 1D Array(array=w550) -> (reversed array=w549:u8[])
      n262 = Reverse 1D Array(array=w577) -> (reversed array=w576:u8[])
      n263 = Reverse 1D Array(array=w584) -> (reversed array=w585:u8[])
      n264 = Reverse 1D Array(array=w571) -> (reversed array=w570:u8[])
      n265 = Reverse 1D Array(array=w541) -> (reversed array=w542:u8[])
      n266 = Type Cast(type=u32 0, x=w600) -> (*(type *) &x=→"GPS1 TOW":u32)
      n267 = Type Cast(type=u32 0, x=w598) -> (*(type *) &x=→"time stamp13":u32)
      n268 = Type Cast(type=u16 0, x=w533) -> (*(type *) &x=w532:u16)
      n269 = Type Cast(type=sgl 0.0, x=w572) -> (*(type *) &x=→"GPS1 VEL E":sgl)
      n270 = Type Cast(type=sgl 0.0, x=w579) -> (*(type *) &x=→"GPS1 VEL N Accuracy":sgl)
      n271 = Type Cast(type=sgl 0.0, x=w582) -> (*(type *) &x=→"GPS1 VEL E Accuracy":sgl)
      n272 = Type Cast(type=sgl 0.0, x=w549) -> (*(type *) &x=→"GPS1 Course":sgl)
      n273 = Type Cast(type=sgl 0.0, x=w576) -> (*(type *) &x=→"GPS1 VEL D":sgl)
      n274 = Type Cast(type=sgl 0.0, x=w585) -> (*(type *) &x=→"GPS1 VEL D Accuracy":sgl)
      n275 = Type Cast(type=sgl 0.0, x=w570) -> (*(type *) &x=→"GPS1 VEL N":sgl)
      n276 = Type Cast(type=sgl 0.0, x=w542) -> (*(type *) &x=→"GPS1 Course Accuracy":sgl)
      n277 = Number To Boolean Array(number=w532) -> (Boolean array=w531:bool[])
      n278 = Array Subset(array=w531, index=0, length=6) -> (w526:bool[])
      n279 = Array Subset(array=w531, index=6, length=6) -> (w525:bool[])
      n280 = Boolean Array To Number(Boolean array=w525) -> (number=w514:u32)
      n281 = Boolean Array To Number(Boolean array=w526) -> (number=w517:u32)
      n282 = node(0 ("key"), "Valid Solution" ("value"), 1 ("value"), "Insufficient SV" ("key"), 2 ("value"), "Internal Error" ("key"), 3 ("value"), "Velocity Limit Excedded" ("key")) -> (w524:map{i32, string})
      n283 = Look In Map(map=w524, key=w517) -> (value=→"GPS1 Velocity Status":string)  [unwired: 1 in, 1 out]
      n284 = node(0 ("key"), "NO Solution" ("value"), 1 ("value"), "Unknown Type" ("key"), 2 ("value"), "Doppler" ("key"), 3 ("value"), "Differential" ("key")) -> (w505:map{i32, string})
      n285 = Look In Map(map=w505, key=w514) -> (value=→"GPS1 Velocity Type":string)  [unwired: 1 in, 1 out]
    }
    frame 14 {
      n286 = Array Subset(array=w610, index=36, length=4) -> (w703:u8[])
      n287 = Array Subset(array=w610, index=40, length=4) -> (w699:u8[])
      n288 = Array Subset(array=w610, index=48, length=4) -> (w712:u8[])
      n289 = Array Subset(array=w610, index=8, length=4) -> (w691:u8[])
      n290 = Array Subset(array=w610, index=28, length=8) -> (w704:u8[])
      n291 = Array Subset(array=w610, index=44, length=4) -> (w698:u8[])
      n292 = Array Subset(array=w610, index=0, length=4) -> (w693:u8[])
      n293 = Array Subset(array=w610, index=12, length=8) -> (w709:u8[])
      n294 = Array Subset(array=w610, index=52, length=1) -> (w717:u8[])
      n295 = Array Subset(array=w610, index=4, length=4) -> (w694:u8[])
      n296 = Array Subset(array=w610, index=54, length=2) -> (w618:u8[])
      n297 = Array Subset(array=w610, index=20, length=8) -> (w706:u8[])
      n298 = Array Subset(array=w610, index=54, length=2) -> (w615:u8[])
      n299 = Reverse 1D Array(array=w694) -> (reversed array=w719:u8[])
      n300 = Reverse 1D Array(array=w691) -> (reversed array=w690:u8[])
      n301 = Reverse 1D Array(array=w693) -> (reversed array=w692:u8[])
      n302 = Reverse 1D Array(array=w706) -> (reversed array=w708:u8[])
      n303 = Reverse 1D Array(array=w703) -> (reversed array=w702:u8[])
      n304 = Reverse 1D Array(array=w699) -> (reversed array=w700:u8[])
      n305 = Reverse 1D Array(array=w712) -> (reversed array=w713:u8[])
      n306 = Reverse 1D Array(array=w704) -> (reversed array=w705:u8[])
      n307 = Reverse 1D Array(array=w698) -> (reversed array=w697:u8[])
      n308 = Reverse 1D Array(array=w709) -> (reversed array=w710:u8[])
      n309 = Reverse 1D Array(array=w717) -> (reversed array=w716:u8[])
      n310 = Reverse 1D Array(array=w618) -> (reversed array=w619:u8[])
      n311 = Reverse 1D Array(array=w615) -> (reversed array=w614:u8[])
      n312 = Type Cast(type=u32 0, x=w690) -> (*(type *) &x=→"GPS1 POS TOW":u32)
      n313 = Type Cast(type=u32 0, x=w692) -> (*(type *) &x=→"time stamp14":u32)
      n314 = Type Cast(type=u32 0, x=w719) -> (*(type *) &x=w601:u32)
      n315 = Number To Boolean Array(number=w601) -> (Boolean array=w605:bool[])
      n316 = Delete From Array(array=w605, length=12, index=0) -> (array with subset deleted=w604:bool[])  [unwired: 1 out]
      n317 = Array To Cluster(array=w604) -> (cluster=→"GPS1 Status":T20)
      n318 = Type Cast(type=0.0, x=w708) -> (*(type *) &x=→"GPS1 Longitude":dbl)
      n319 = Type Cast(type=sgl 0.0, x=w702) -> (*(type *) &x=w607:sgl)
      "GPS1 Undulation" <- w607
      n320 = Type Cast(type=sgl 0.0, x=w700) -> (*(type *) &x=→"GPS1 Latitude Accuracy":sgl)
      n321 = Type Cast(type=sgl 0.0, x=w713) -> (*(type *) &x=→"GPS1 Altitude Accuracy":sgl)
      n322 = Type Cast(type=0.0, x=w705) -> (*(type *) &x=w608:dbl)
      "GPS1 Altitude MSL" <- w608
      n323 = Type Cast(type=sgl 0.0, x=w697) -> (*(type *) &x=→"GPS1 Longitude Accuracy":sgl)
      n324 = Type Cast(type=0.0, x=w710) -> (*(type *) &x=→"GPS1 Latitude":dbl)
      n325 = Type Cast(type=u8 0, x=w716) -> (*(type *) &x=→"GPS1 SV_NUM":u8)
      n326 = Type Cast(type=u16 0, x=w619) -> (*(type *) &x=→"GPS1 Base Station ID":u16)
      n327 = Type Cast(type=u16 0, x=w614) -> (*(type *) &x=→"GPS1 Differential Data age":u16)
      n328 = Number To Boolean Array(number=w601) -> (Boolean array=w720:bool[])
      n329 = Array Subset(array=w720, index=6, length=6) -> (w722:bool[])
      n330 = Array Subset(array=w720, index=0, length=6) -> (w721:bool[])
      n331 = Add(x=w608, y=w607) -> (x+y=→"GPS1 Altitude WGS-84 2":dbl)
      n332 = Boolean Array To Number(Boolean array=w722) -> (number=w727:u32)
      n333 = Boolean Array To Number(Boolean array=w721) -> (number=w724:u32)
      n334 = node(0 ("key"), "Valid Solution" ("value"), 1 ("value"), "Insufficient SV" ("key"), 2 ("value"), "Internal Error" ("key"), 3 ("value"), "Height Limit Excedded" ("key")) -> (w723:map{i32, string})
      n335 = Look In Map(map=w723, key=w724) -> (value=→"GPS1 POS Status":string)  [unwired: 1 in, 1 out]
      n336 = node(0 ("key"), "NO Solution" ("value"), 1 ("value"), "Unknown Type" ("key"), 2 ("value"), "Single Point" ("key"), 3 ("value"), "DGPS" ("key"), 4 ("key"), "SBAS sat. Used" ("value"), 5 ("key"), "Omnistar VBS Position (L1 sub-meter)" ("value"), 6 ("key"), "Floating RTK ambiguity solution (20 cms RTK)" ("value"), 7 ("key"), "Integer RTK ambiguity solution (2 cms RTK)" ("value"), 8 ("key"), "Precise Point Positioning with float ambiguities" ("value"), 9 ("key"), "T Precise Point Positioning with fixed ambiguities" ("value"), 10 ("key"), "Fixed location solution position" ("value")) -> (w728:map{i32, string})
      n337 = Look In Map(map=w728, key=w727) -> (value=→"GPS1 POS Type":string)  [unwired: 1 in, 1 out]
    }
  }
  n338 = local read "Vertical velocity (positive down)"() -> (w1:sgl)
  n339 = local read "Pitch"() -> (w17:sgl)
  n340 = local read "Roll"() -> (w19:sgl)
  n341 = local read "Yaw"() -> (w16:sgl)
  n342 = local read "EKF Altitude MSL"() -> (w20:dbl)
  n343 = local read "GPS1 Altitude MSL"() -> (w28:dbl)
  n344 = local read "EKF Longitude"() -> (w21:dbl)
  n345 = local read "GPS1 Longitude"() -> (w29:dbl)
  n346 = local read "EKF Latitude"() -> (w22:dbl)
  n347 = local read "GPS1 Latitude"() -> (w30:dbl)
  n348 = local read "GPS1 SV_NUM"() -> (w24:u8)
  n349 = local read "time stamp01"() -> (w25:u32)
  n350 = local read "GPS1 Course"() -> (w31:sgl)
  n351 = local read "GPS1 TOW"() -> (w23:u32)
  n352 = local read "Up Time"() -> (w26:u32)
  n353 = expression code="(x/pi)*180.0" "radians to degrees"(w19) -> (w18:sgl)
  n354 = expression code="(x/pi)*180.0" "radians to degrees"(w17) -> (w15:sgl)
  n355 = expression code="(x/pi)*180.0" "radians to degrees"(w16) -> (w14:sgl)
  n356 = Bundle By Name(cluster=T1 {"Up Time"=0, "Timestamp"=0, "Yaw"=0.0, "Pitch"=0.0, "Roll"=0.0, "EKF Lat"=0.0, "EKF Lon"=0.0, "EKF Alt"=0.0, "GPS Lat"=0.0, "GPS Lon"=0.0, "GPS Alt"=0.0, "GPS Course"=0.0, "GPS SV Num"=0, "GPS TOW"=0, "Vert Speed"=0.0} ("SBG Data Cluster"), "Up Time"=w26, "Timestamp"=w25, "Roll"=w18, "Pitch"=w15, "Yaw"=w14, "GPS Course"=w31, "GPS Lat"=w30, "GPS Lon"=w29, "GPS Alt"=w28, "GPS SV Num"=w24, "GPS TOW"=w23, "EKF Lat"=w22, "EKF Lon"=w21, "EKF Alt"=w20, "Vert Speed"=w1) -> (w6:T1)
  "output cluster" <- w6
  n357 = call "Compass.vi"("GPS/Mag"=TRUE, "SBG Data Cluster"=w6) -> ("Heading Digital"=→"Heading Digital":dbl, "CompassGauge"=→"CompassGauge":picture)  [unwired: 7 in, 1 out]
  n358 = call "ArtificialHorizon.vi"("SBG Data Cluster"=w6) -> ("ArtificialHorizon"=→"ArtificialHorizon":picture)  [unwired: 9 in, 1 out]
  n359 = call "AltitudeIndicator.vi"("SBG Data Cluster"=w6, "ScaleUnit(F=m; T=feet)"="ScaleUnit(F=m; T=feet)") -> ("Altitude  (/10000)"=→"Altitude  (/10000)":dbl, "AltitudeIndicator"=→"AltitudeIndicator":picture)  [unwired: 5 in, 3 out]
  n360 = call "VerticalSpeedIndicator.vi"("SignalSource"=T12."Baro Vario", "ScaleUnit(F=m/s; T=Ft/min/100)"=FALSE, "SBG Data Cluster"=w6) -> ("VerticalSpeedDigital"=→"VerticalSpeedDigital":dbl, "VerticalSpeedIndicator"=→"VerticalSpeedIndicator":picture)  [unwired: 6 in, 1 out]
